vi "Keithley24XX_SR830_LakeShore336_4Probe_Resistance_Measurement_v3_Sequential.vi"() -> ()   [LabVIEW 2020]
uses:
  instr.lib/Lake Shore 336/Public/Data/Sensor Data (Single Reading).vi
  instr.lib/Stanford Research 830/Public/Data/Read (All Parameters).vi
  instr.lib/Keithley 24XX/Public/Data/Read (Single Point).vi
  instr.lib/Keithley 24XX/Keithley 24XX.lvlib
  instr.lib/Stanford Research 830/Stanford Research 830.lvlib
  instr.lib/Lake Shore 336/Lake Shore 336.lvlib
panel:
  out "Denumerated Sense":dbl
  out "SR830 X-Value":dbl
  out "SR830 Theta-Value":dbl
  out "Live Sensitivity":i16(ring)=17 items=["Auto Gain"=-1, "2 nV/fA"=0, "5 nV/fA"=1, "10 nV/fA"=2, "20 nV/fA"=3, "50 nV/fA"=4, "100 nV/fA"=5, "200 nV/fA"=6, "500 nV/fA"=7, "1 uV/pA"=8, "2 uV/pA"=9, "5 uV/pA"=10, "10 uV/pA"=11, "20 uV/pA"=12, "50 uV/pA"=13, "100 uV/pA"=14, "200 uV/pA"=15, "500 uV/pA"=16, "1 mV/nA"=17, "2 mV/nA"=18, "5 mV/nA"=19, "10 mV/nA"=20, "20 mV/nA"=21, "50 mV/nA"=22, "100 mV/nA"=23, "200 mV/nA"=24, "500 mV/mA"=25, "1 V/uA"=26]
  in  "Sensitivity (Initial Value)":i16(ring)=17 items=["Auto Gain"=-1, "2 nV/fA"=0, "5 nV/fA"=1, "10 nV/fA"=2, "20 nV/fA"=3, "50 nV/fA"=4, "100 nV/fA"=5, "200 nV/fA"=6, "500 nV/fA"=7, "1 uV/pA"=8, "2 uV/pA"=9, "5 uV/pA"=10, "10 uV/pA"=11, "20 uV/pA"=12, "50 uV/pA"=13, "100 uV/pA"=14, "200 uV/pA"=15, "500 uV/pA"=16, "1 mV/nA"=17, "2 mV/nA"=18, "5 mV/nA"=19, "10 mV/nA"=20, "20 mV/nA"=21, "50 mV/nA"=22, "100 mV/nA"=23, "200 mV/nA"=24, "500 mV/mA"=25, "1 V/uA"=26]
  in  "Dynamic Reserve (-1 = Auto)":i16(ring)=-1 items=["Auto Reserve"=-1, "High Reserve"=0, "Normal"=1, "Low Noise"=2]
  in  "Input Connection (0: Single-Ended Voltage)":u16(ring)=1 items=["Single-Ended Voltage", "Differential Voltage", "1 MOhm Current Gain", "100 MOhm Current Gain"]
  out "Input Coupling (0: AC)":u16(ring) items=["AC", "DC"]
  in  "Time Constant (8: 100ms)":u16(ring)=9 items=["10 us", "30 us", "100 us", "300 us", "1 ms", "3 ms", "10 ms", "30 ms", "100 ms", "300 ms", "1 s", "3 s", "10 s", "30 s", "100 s", "300 s", "1 ks", "3 ks", "10 ks", "30 ks"]
  in  "SR830 VISA resource name":refnum<visa-resource-name>="GPIB0::10::INSTR"
  out "Sense\nUnder":bool
  out "Sense\nOver":bool
  in  "Trigger Source (0: Internal)":u16(ring) items=["Internal", "External"]
  out "Manual Phase (0 Degree)":dbl
  out "Detection Harmonic Number":dbl=1.0
  out "External Reference Trigger (0: Sine Zero Crossing)":u16(ring) items=["Sine Zero Crossing", "TTL Rising Edge", "TTL Falling Edge"]
  in  "Internal Reference Frequency (1000 Hz)":dbl=17.0
  in  "Reference Source (1: Internal)":u16(ring)=1 items=["External", "Internal"]
  in  "Sine Output Amplitude (V)":dbl=1.0
  out "Gate\nVoltage":sgl
  out "Status":sgl
  out "Leakage \nCurrent":sgl
  in  "Temp Vs Time":enum32{"XY Graph", "Waveform (Time)"}(tab)
  out "Temp vs Time : XYGraph":cluster{"Y":dbl[], "Y":dbl[]}[](graph)
  out "Temp vs Time : TimeGraph":cluster{i32, "Sensor Data":dbl}[](graph)
  in  "Data Source (0:Kelvin)":u16(ring) items=["Kelvin", "Celsius", "Sensor Units"]
  in  "Input (0:A)":u16(ring) items=["A", "B", "C", "D"]
  in  "Serial Configuration 2":T1={"Baud Rate"=57600, "Parity"=1, "Data Bits"=7, "Stop Bits"=10, "Flow Control"=0} {"Flow Control" items=["None", "XON/XOFF", "RTS/CTS", "XON/XOFF & RTS/CTS", "DTR/DSR", "XON/XOFF & DTR/DSR"]; "Stop Bits" items=["1.0"=10, "1.5"=15, "2.0"=20]; "Data Bits" items=["7"=7, "8"=8]; "Parity" items=["None", "Odd", "Even", "Mark", "Space"]; "Baud Rate" items=["300"=300, "600"=600, "1200"=1200, "2400"=2400, "4800"=4800, "9600"=9600, "19200"=19200, "38400"=38400, "57600"=57600]}
  in  "LakeShore 336 esource name":refnum<visa-resource-name>="GPIB0::12::INSTR"
  out "dup path":path
  in  "<File Name>.txt (Don't add extension)":string
  in  "Data Save Path:":path=path "C:/Users/labpc/Documents/ProbeStation Users Data"
  in  "I_leak vs Vg":enum32{"XY Graph", "Waveform (Time)"}(tab)
  out "I_leak vs Vg : XYGraph":cluster{"Y":dbl[], "Y":dbl[]}[](graph)
  out "I_leak vs Vg : TimeGraph":cluster{dbl, "Current":sgl}[](graph)
  in  "Gate Voltage\nInitial (V)":dbl
  out "Gate Voltage\nTraversal Direction":enum16{"Upward", "Downward"}(ring)
  in  "Series Resistance \n(Apparatus Constant)":dbl=10000000.0
  in  "stop":bool
  out "Max/Min(-) \nGate Voltage (V)":dbl=80.0
  in  "Gate Voltage \nStep Size (V)":dbl=0.1
  in  "High Gate \nVoltage (V)":dbl
  in  "Low Gate \nVoltage (V)":dbl
  out "Compliance\n Level (A)":dbl=0.1
  in  "Theta vs Vg":enum32{"XY Graph", "Waveform (Time)"}(tab)
  out "Theta vs Vg : XYGraph":cluster{"Y":dbl[], "Y":dbl[]}[](graph)
  out "Theta vs Vg : TimeGraph":cluster{dbl, "Theta-Value":dbl}[](graph)
  in  "R vs Vg":enum32{"XY Graph", "Waveform (Time)"}(tab)
  out "Resistance vs Vg : XYGraph":cluster{"Y":dbl[], "Y":dbl[]}[](graph)
  out "R vs Vg : TimeGraph":cluster{dbl, dbl}[](graph)
  in  "Serial Configuration":T1={"Baud Rate"=9600, "Parity"=0, "Data Bits"=8, "Stop Bits"=10, "Flow Control"=0} {"Flow Control" items=["None", "XON/XOFF", "RTS/CTS", "XON/XOFF & RTS/CTS", "DTR/DSR", "XON/XOFF & DTR/DSR"]; "Stop Bits" items=["1.0"=10, "1.5"=15, "2.0"=20]; "Data Bits" items=["7"=7, "8"=8]; "Parity" items=["None", "Odd", "Even", "Mark", "Space"]; "Baud Rate" items=["300"=300, "600"=600, "1200"=1200, "2400"=2400, "4800"=4800, "9600"=9600, "19200"=19200]}
  in  "Keithley24XX VISA resource name":refnum<visa-resource-name>="GPIB0::21::INSTR" caption="Keithley 24XX VISA resource name"
  out "Internal Delay\nMeasurement Time (S)":dbl
  # "Lake Shore 336 Temp Contr."
  # "SR830 Lock In Amplifier"
  # "MAKE SURE THE SOURCE METER IS ON TO ENSURE NO UNINTENDED JUMPS. PROGRAM WILL KEEP SOURCE METER ON ONCE RUN."
  # "Keithley 2400 SourceMeter"
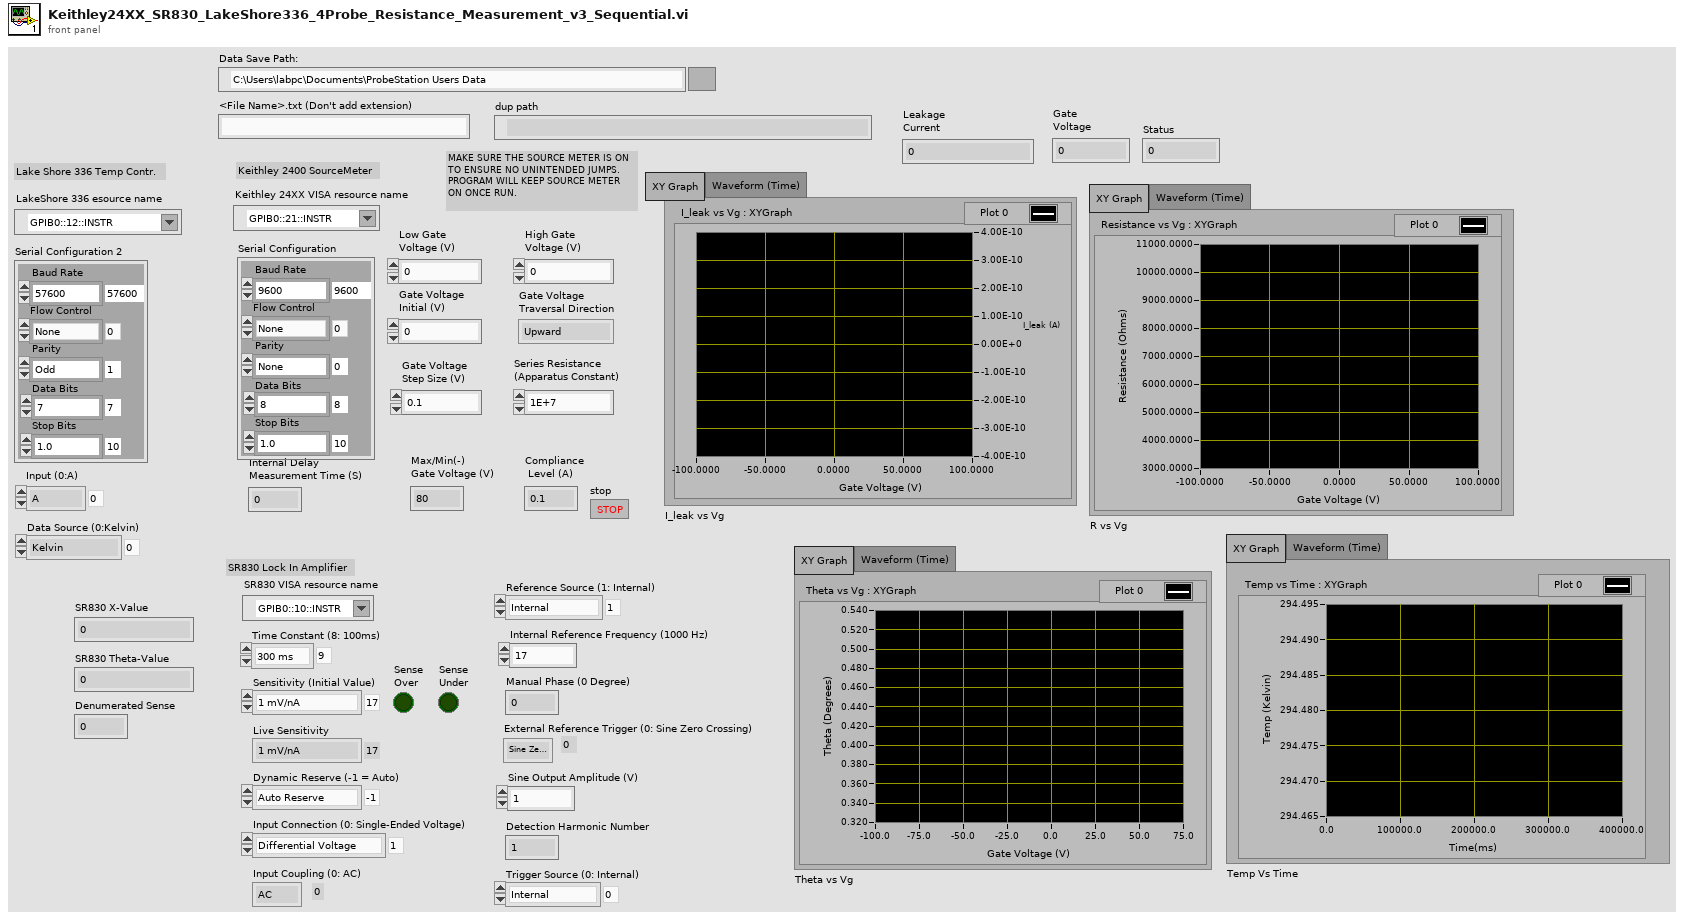
[diagram p1: front panel]
types:
  T1 = cluster{"Baud Rate":u32, "Parity":u16, "Data Bits":u16, "Stop Bits":u16, "Flow Control":u16}
  T2 = enum16{"open", "replace", "create", "open or create", "replace or create", "replace or create with confirmation"}
  T3 = cluster{"X-Value":dbl, "Y-Value":dbl, "R-Value":dbl, "Theta-Value":dbl, "Aux In 1 Value":dbl, "Aux In 2 Value":dbl, "Aux In 3 Value":dbl, "Aux In 4 Value":dbl, "Reference Frequency":dbl, "Channel 1 Display":dbl, "Channel 2 Display":dbl}
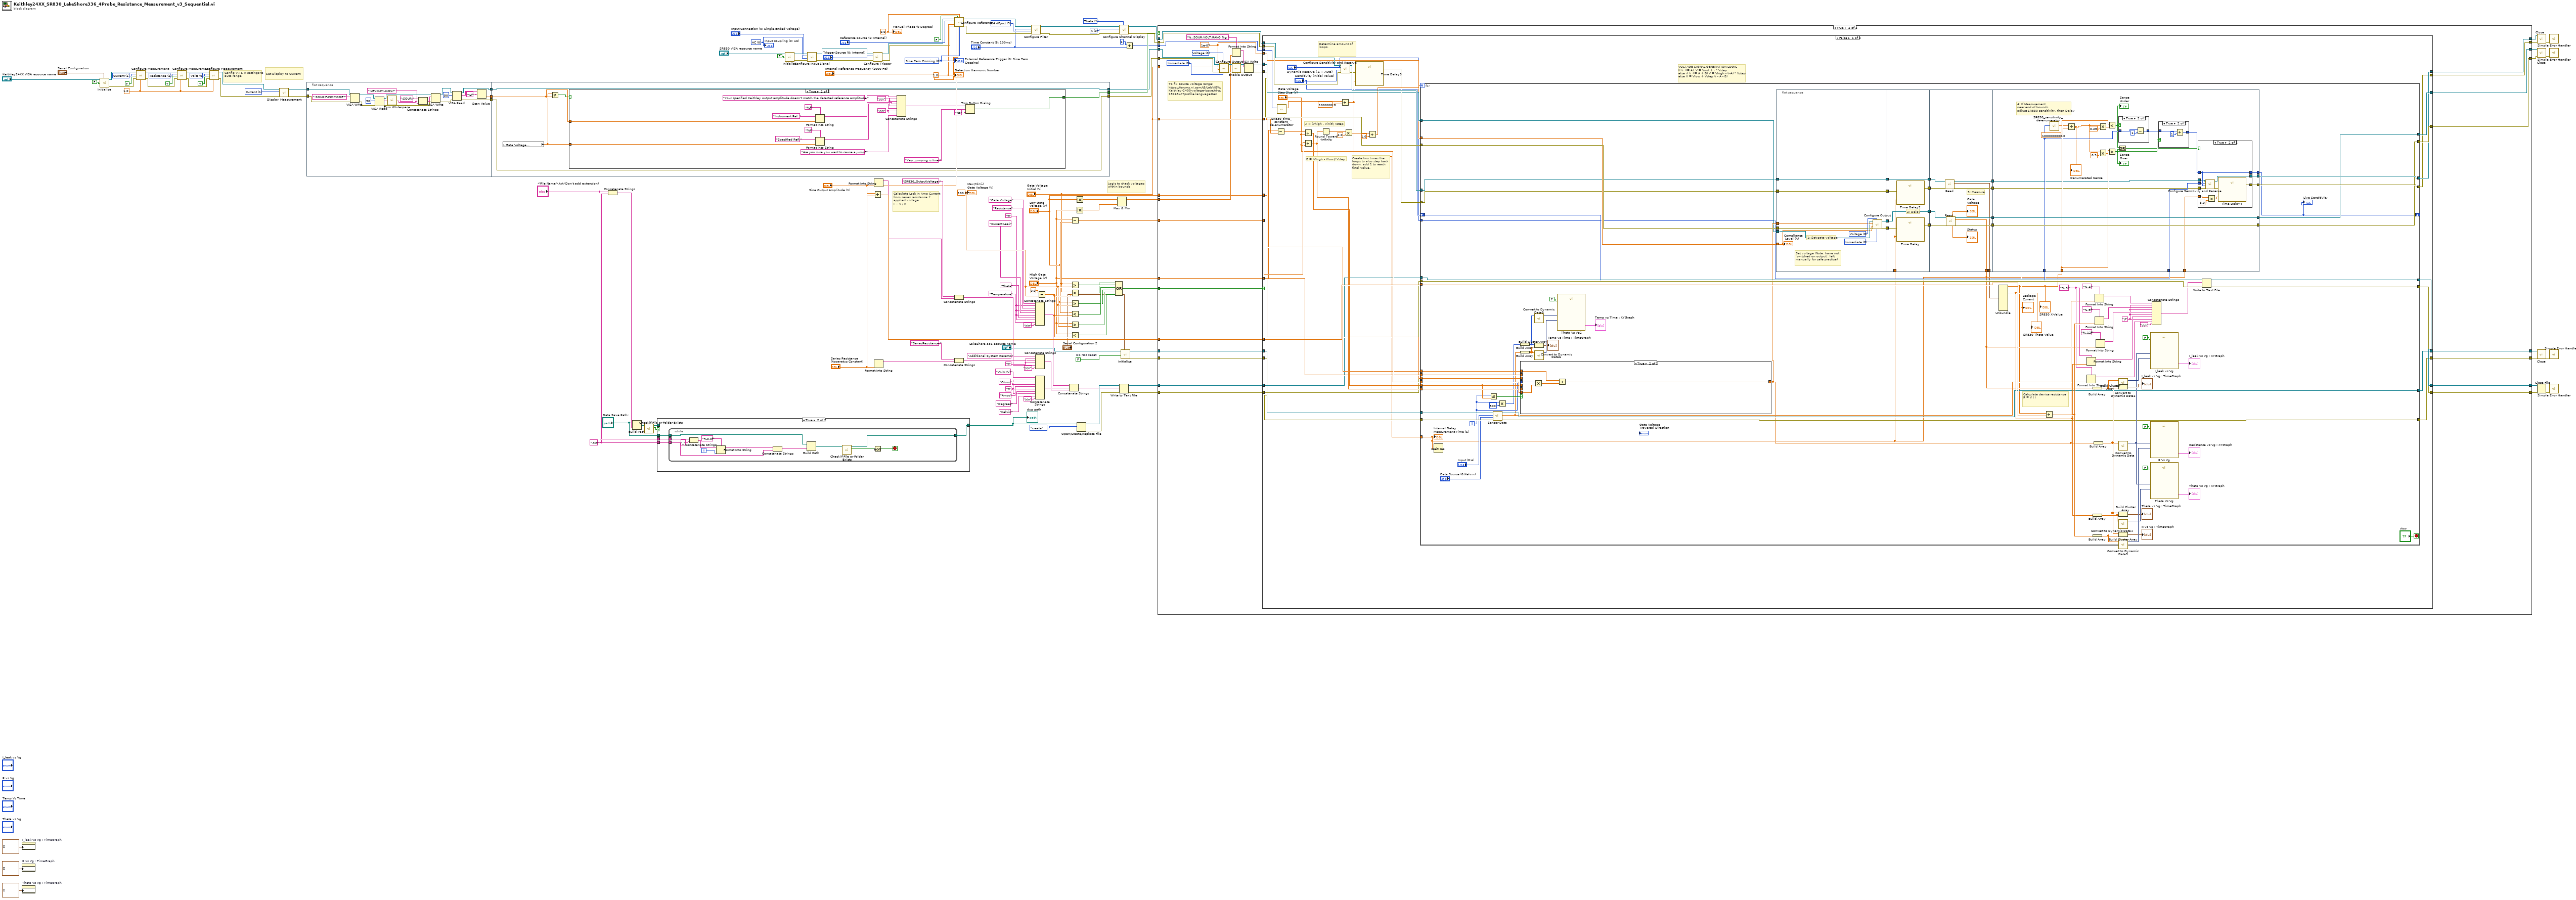
[diagram p0: block diagram]
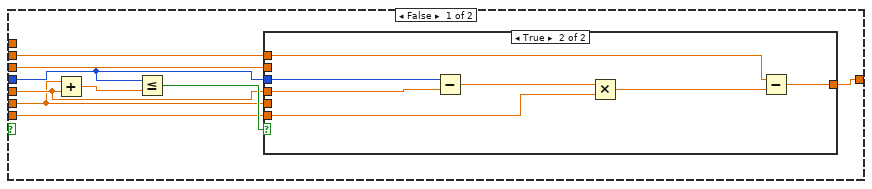
[diagram p6: hidden frame]
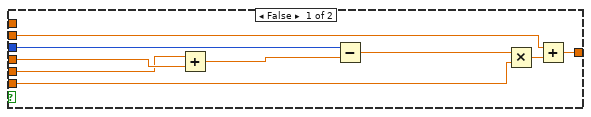
[diagram p7: hidden frame]
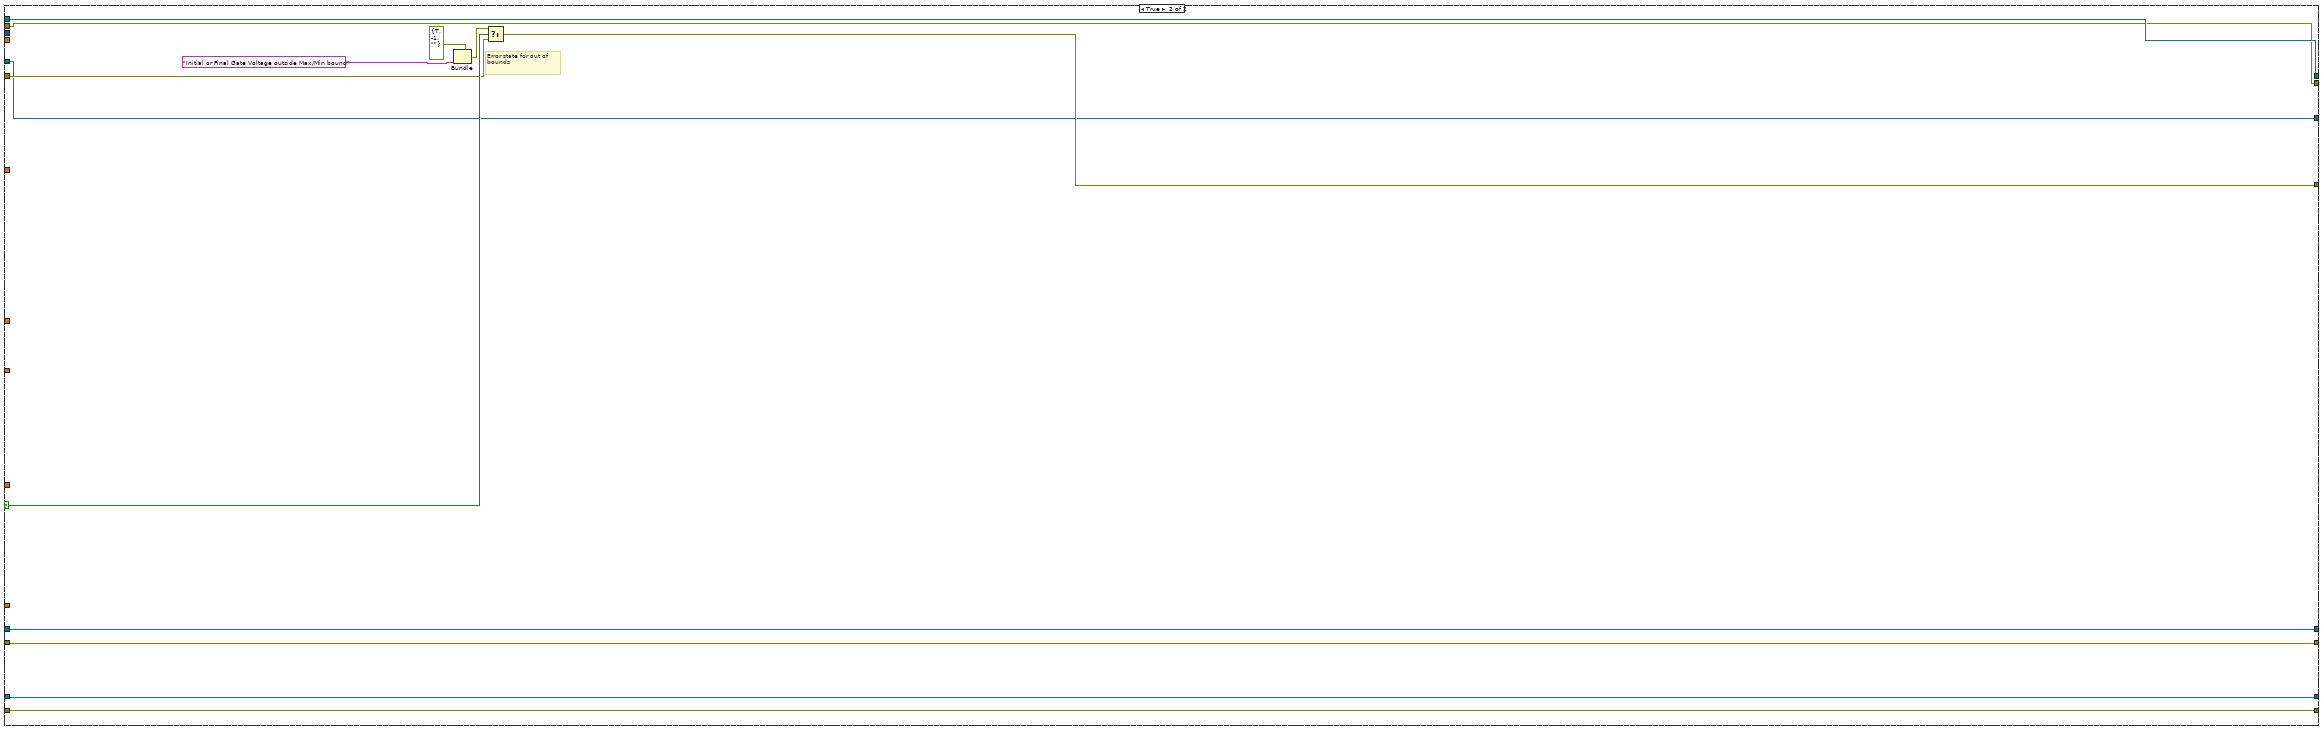
[diagram p8: hidden frame]
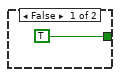
[diagram p9: hidden frame]
diagram:
  w4 = u16 3 items=["6 dB/oct", "12 dB/oct", "18 db/oct", "24 dB/oct"] ("Low Pass Filter Slope (1: 12dB/oct)")
  w31 = FALSE  # Do Not Reset
  w37 = "\t"
  w20 = "\t"
  w22 = "\t"
  w65 = ".txt"
  w72 = 1.0 ("Manual Range (1.0)")
  w96 = 0.0 ("Manual Phase (0 Degree)")
  w97 = 1.0 ("Detection Harmonic Number (1)")
  w98 = u16 0 items=["Sine Zero Crossing", "TTL Rising Edge", "TTL Falling Edge"] ("External Reference Trigger (0: Sine Zero Crossing)")
  w102 = u16 0 items=["AC", "DC"] ("Input Coupling (0: AC)")
  w84 = u16 0 items=["X", "R", "X Noise", "Aux In 1", "Aux In 2"] ("Channel 1 Display (0: X)")
  w111 = u16 1 items=["Y", "Theta", "Y Noise", "Aux In 3", "Aux In 4"] ("Channel 2 Display  (0: Y)")
  w116 = u16 1 items=["Voltage", "Current", "Resistance"] ("Displayed Measurement (0: Voltage)")
  w125 = u16 2 items=["Volts", "Current", "Resistance"] ("Function (0: Volts)")
  w129 = u16 1 items=["Volts", "Current", "Resistance"] ("Function (0: Volts)")
  w73 = 100.0
  w135 = u16 0 items=["Volts", "Current", "Resistance"] ("Function (0: Volts)")
  # "Logic to check voltages within bounds"
  # "Calculate Lock In Amp Current from series resistance + applied voltage\nI = V / R"
  # "Set Display to Current"
  # "Config V,I & R settings to auto range"
  n1 = property on="I_leak vs Vg : TimeGraph" class="WFChart (strict)"("History Data"=cluster{dbl, "Current":sgl}[] []) -> ()  [unwired: 2 in, 2 out]
  n2 = property on="R vs Vg : TimeGraph" class="WFChart (strict)"("History Data"=cluster{dbl, dbl}[] []) -> ()  [unwired: 2 in, 2 out]
  n3 = property on="Theta vs Vg : TimeGraph" class="WFChart (strict)"("History Data"=cluster{dbl, "Theta-Value":dbl}[] []) -> ()  [unwired: 2 in, 2 out]
  n4 = call "Initialize.vi"("Serial Configuration"="Serial Configuration", "Reset (True)"=FALSE, "VISA resource name"="Keithley24XX VISA resource name") -> ("error out"=w120:errorcluster, "VISA resource name out"=w121:refnum<visa-resource-name>)  [unwired: 7 in]
  n5 = call "Configure Measurement.vi"("Manual Range (1.0)"=w72, "error in (no error)"=w120, "Enable Auto Range (T:Enable)"=TRUE, "Function (0: Volts)"=w129, "VISA resource name"=w121) -> ("error out"=w127:errorcluster, "VISA resource name out"=w122:refnum<visa-resource-name>)  [unwired: 5 in]
  n6 = call "Configure Measurement.vi"("Manual Range (1.0)"=w72, "error in (no error)"=w127, "Enable Auto Range (T:Enable)"=TRUE, "Function (0: Volts)"=w125, "VISA resource name"=w122) -> ("error out"=w124:errorcluster, "VISA resource name out"=w123:refnum<visa-resource-name>)  [unwired: 5 in]
  n7 = call "Configure Measurement.vi"("Manual Range (1.0)"=w72, "error in (no error)"=w124, "Enable Auto Range (T:Enable)"=TRUE, "Function (0: Volts)"=w135, "VISA resource name"=w123) -> ("error out"=w114:errorcluster, "VISA resource name out"=w115:refnum<visa-resource-name>)  [unwired: 5 in]
  n8 = call "Display Measurement.vi"("error in (no error)"=w114, "Displayed Measurement (0: Voltage)"=w116, "VISA resource name"=w115) -> ("error out"=w10:errorcluster, "VISA resource name out"=w11:refnum<visa-resource-name>)  [unwired: 7 in]
  n9 = flat-sequence {
    tunnel: [w139] -> w14
    tunnel: [w140] -> w13
    tunnel: [w141] -> w12
    tunnel: w11 -> [w138]
    tunnel: w10 -> [w137]
    tunnel: w14 -> [w160]
    tunnel: w13 -> [w159]
    tunnel: w12 -> [w163]
    tunnel: [w160] -> w6
    tunnel: [w159] -> w8
    tunnel: [w158] -> w9
    frame #0 {
      n10 = VISA Write(VISA resource name=w138, write buffer=":SOUR:FUNC:MODE?", error in (no error)=w137) -> (VISA resource name out=w154:refnum<visa-resource-name>, error out=w157:errorcluster)  [unwired: 1 out]
      n11 = VISA Read(VISA resource name=w154, byte count=u32 50, error in (no error)=w157) -> (VISA resource name out=w149:refnum<visa-resource-name>, read buffer=w143:string, error out=w150:errorcluster)  [unwired: 1 out]
      n12 = call <vilib>:"Trim Whitespace.vi"("string"=w143) -> ("trimmed string"=w142:string)  [unwired: 1 in]
      n13 = Concatenate Strings(":SOUR:" ("string"), w142, ":LEV:IMM:AMPL?" ("string")) -> (w146:string)
      n14 = VISA Write(VISA resource name=w149, write buffer=w146, error in (no error)=w150) -> (VISA resource name out=w151:refnum<visa-resource-name>, error out=w153:errorcluster)  [unwired: 1 out]
      n15 = VISA Read(VISA resource name=w151, byte count=u32 50, error in (no error)=w153) -> (VISA resource name out=w139:refnum<visa-resource-name>, read buffer=w144:string, error out=w140:errorcluster)  [unwired: 1 out]
      n16 = Scan Value(string=w144, format string="%f") -> (value=w141:dbl)  [unwired: 1 in, 1 out]
    }
    frame #1 {
      n17 = local read "Gate Voltage\nInitial (V)"() -> (w161:dbl)
      n18 = Not Equal?(x=w161, y=w163) -> (x != y?=w162:bool)
      n19 = case shown="True" w162 {
        tunnel: [TRUE ("T button?") w171] -> w158
        tunnel: w163 -> [_ w166]
        tunnel: w161 -> [_ w165]
        frame False {
        }
        frame True {
          w169 = "\r\n"
          w167 = "\r\n"
          n20 = Format Into String(format string="%f", initial string="Instrument Ref: ", w166) -> (resulting string=w173:string)  [unwired: 1 in, 1 out]
          n21 = Format Into String(format string="%f", initial string="Specified Ref: ", w165) -> (resulting string=w172:string)  [unwired: 1 in, 1 out]
          n22 = Concatenate Strings("Your specified Keithley output amplitude doesn't match the detected reference amplitude." ("message"), w167, w167, w173, w167, w172, w169, w169, "Are you sure you want to cause a jump?" ("string")) -> (w178:string)
          n23 = Two Button Dialog(message=w178, 1:"No" ("F button name (\"Cancel\")"), 2:"Yep, jumping is fine." ("T button name (\"OK\")")) -> (T button?=w171:bool)
        }
      }
    }
  }
  n24 = Concatenate Strings("<File Name>.txt (Don't add extension)", w65) -> (w71:string)
  n25 = Build Path(base path="Data Save Path:", name or relative path=w71) -> (appended path=w70:path)
  n26 = call <vilib>:"Check if File or Folder Exists.vi"("path"=w70) -> ("file or folder exists?"=w69:bool, "dup path"=w68:path)  [unwired: 8 in, 1 out]
  n27 = case shown="True" w69 {
    tunnel: [w181 w182] -> w62
    tunnel: w68 -> [w181 _]
    tunnel: "Data Save Path:" -> [_ w183]
    tunnel: "<File Name>.txt (Don't add extension)" -> [_ w185]
    tunnel: w65 -> [_ w184]
    frame False {
    }
    frame True {
      n28 = while {
        tunnel: w185 -> [w188]
        tunnel: w184 -> [w193]
        tunnel: w183 -> [w191]
        tunnel: [w189] -> w182
        i -> [w195]
        stop <- w197 stop-if-true
        n29 = Concatenate Strings(w188, "_" ("string")) -> (w187:string)
        n30 = Format Into String(format string="%0.0f", initial string=w187, w195) -> (resulting string=w194:string)  [unwired: 1 in, 1 out]
        n31 = Concatenate Strings(w194, w193) -> (w192:string)
        n32 = Build Path(base path=w191, name or relative path=w192) -> (appended path=w190:path)
        n33 = call <vilib>:"Check if File or Folder Exists.vi"("path"=w190) -> ("file or folder exists?"=w198:bool, "dup path"=w189:path)  [unwired: 8 in, 1 out]
        n34 = Not(x=w198) -> (.not. x?=w197:bool)
      }
    }
  }
  "dup path" <- w62
  n35 = call "Initialize.vi"("Reset (True)"=FALSE, "VISA resource name"="SR830 VISA resource name") -> ("error out"=w109:errorcluster, "VISA resource name out"=w110:refnum<visa-resource-name>)  [unwired: 8 in]
  n36 = call "Configure Input Signal.vi"("error in (no error)"=w109, "Input Coupling (0: AC)"=w102, "Input Connection (0: Single-Ended Voltage)"="Input Connection (0: Single-Ended Voltage)", "VISA resource name"=w110) -> ("error out"=w93:errorcluster, "VISA resource name out"=w94:refnum<visa-resource-name>)  [unwired: 6 in]
  n37 = call "Configure Trigger.vi"("error in (no error)"=w93, "Trigger Source (0: Internal)"="Trigger Source (0: Internal)", "VISA resource name"=w94) -> ("error out"=w91:errorcluster, "VISA resource name out"=w92:refnum<visa-resource-name>)  [unwired: 7 in]
  n38 = Divide(x="Sine Output Amplitude (V)", y="Series Resistance \n(Apparatus Constant)") -> (x/y=w90:dbl)
  n39 = Format Into String("Sine Output Amplitude (V)") -> (resulting string=w54:string)  [unwired: 3 in, 1 out]
  n40 = Format Into String("Series Resistance \n(Apparatus Constant)") -> (resulting string=w55:string)  [unwired: 3 in, 1 out]
  n41 = call "Configure Reference.vi"("VISA resource name"=w92, "Auto Phase (T: Enabled)"=FALSE, "Manual Phase (0 Degree)"=w96, "Reference Source (1: Internal)"="Reference Source (1: Internal)", "Sine Output Amplitude (1 V)"="Sine Output Amplitude (V)", "Detection Harmonic Number (1)"=w97, "error in (no error)"=w91, "Internal Reference Frequency (1000 Hz)"="Internal Reference Frequency (1000 Hz)", "External Reference Trigger (0: Sine Zero Crossing)"=w98) -> ("VISA resource name out"=w99:refnum<visa-resource-name>, "error out"=w100:errorcluster)  [unwired: 5 in]
  n42 = Concatenate Strings("SR830_OutputVoltage:" ("string"), w54) -> (w35:string)
  n43 = Concatenate Strings("SeriesResistance:" ("string"), w55) -> (w36:string)
  n44 = call "Configure Filter.vi"("error in (no error)"=w100, "Low Pass Filter Slope (1: 12dB/oct)"=w4, "Time Constant (8: 100ms)"="Time Constant (8: 100ms)", "VISA resource name"=w99) -> ("error out"=w118:errorcluster, "VISA resource name out"=w117:refnum<visa-resource-name>)  [unwired: 6 in]
  n45 = Concatenate Strings("Gate Voltage" ("string"), w22, "Resistance" ("string"), w22, "Current Leak" ("string"), w22, "Theta" ("string"), w22, "Temperature" ("string"), "\r\n") -> (w49:string)
  n46 = Concatenate Strings("Volts (V)" ("string"), w20, "Ohms" ("string"), w20, "Amps" ("string"), w20, "Degrees" ("string"), w20, "Kelvin" ("string"), "\r\n") -> (w48:string)
  n47 = Concatenate Strings("Additional System Params:" ("string"), w37, w36, w37, w35, "\r\n") -> (w38:string)
  n48 = Subtract(x=0.0, y=w73) -> (x-y=w78:dbl)
  n49 = Concatenate Strings(w49, w48, w38) -> (w33:string)
  n50 = Subtract(x="High Gate \nVoltage (V)", y="Low Gate \nVoltage (V)") -> (x-y=w74:dbl)
  n51 = Greater?(x="Gate Voltage\nInitial (V)", y=w73) -> (0:w77:bool)
  n52 = Less?(x="Gate Voltage\nInitial (V)", y=w78) -> (x < y?=w76:bool)
  n53 = Greater?(x="Low Gate \nVoltage (V)", y=w73) -> (0:w81:bool)
  n54 = Less?(x="Low Gate \nVoltage (V)", y=w78) -> (x < y?=w82:bool)
  n55 = Greater?(x="High Gate \nVoltage (V)", y=w73) -> (0:w80:bool)
  n56 = Less?(x="High Gate \nVoltage (V)", y=w78) -> (x < y?=w79:bool)
  n57 = Absolute Value(x="Low Gate \nVoltage (V)") -> (abs(x)=w18:dbl)
  n58 = Absolute Value(x="High Gate \nVoltage (V)") -> (abs(x)=w17:dbl)
  n59 = Open/Create/Replace File(file path (use dialog)=w62, operation (0:open)=T2."create") -> (refnum out=w63:refnum<file>, error out=w61:errorcluster)  [unwired: 4 in, 1 out]
  n60 = Compound Arithmetic op=OR(w76, w77, w82, w81, w80, w79) -> (w75:bool)
  n61 = Max & Min(x=w18, y=w17) -> (max(x,y)=w5:dbl)  [unwired: 1 out]
  n62 = Write to Text File(file (use dialog)=w63, text=w33, error in=w61) -> (refnum out=w59:refnum<file>, error out=w58:errorcluster)  [unwired: 1 in, 1 out]
  n63 = call "Configure Channel Display.vi"("Channel 2 Display  (0: Y)"=w111, "error in (no error)"=w118, "Channel 1 Display (0: X)"=w84, "VISA resource name"=w117) -> ("error out"=w107:errorcluster, "VISA resource name out"=w108:refnum<visa-resource-name>)  [unwired: 6 in]
  n64 = call "Initialize.vi"("Serial Configuration"="Serial Configuration 2", "Reset (True)"=w31, "VISA resource name"="LakeShore 336 esource name") -> ("error out"=w26:errorcluster, "VISA resource name out"=w25:refnum<visa-resource-name>)  [unwired: 7 in]
  n65 = Add(x=u16 1, y="Time Constant (8: 100ms)") -> (x+y=w1:u16)
  n66 = case shown="True" w9 {
    tunnel: [w206 w242] -> w133
    tunnel: [w205 w241] -> w132
    tunnel: w108 -> [w204 w240]
    tunnel: w107 -> [w203 w239]
    tunnel: [w204 w238] -> w106
    tunnel: [w203 w237] -> w105
    tunnel: w90 -> [_ w236]
    tunnel: w75 -> [_ w235]
    tunnel: w74 -> [_ w234]
    tunnel: w59 -> [w202 w233]
    tunnel: w58 -> [w201 w232]
    tunnel: [w202 w231] -> w57
    tunnel: [w201 w230] -> w56
    tunnel: [w199 w229] -> w28
    tunnel: [w200 w228] -> w27
    tunnel: w26 -> [w199 w227]
    tunnel: w25 -> [w200 w226]
    tunnel: "Low Gate \nVoltage (V)" -> [_ w225]
    tunnel: "High Gate \nVoltage (V)" -> [_ w224]
    tunnel: "Gate Voltage\nInitial (V)" -> [_ w223]
    tunnel: w8 -> [w205 w215]
    tunnel: "Gate Voltage\nInitial (V)" -> [_ w214]
    tunnel: w6 -> [w206 w213]
    tunnel: w5 -> [_ w211]
    tunnel: w1 -> [_ w207]
    frame False {
    }
    frame True {
      w217 = u16 0 items=["Immediate", "Triggered"] ("Output Type  (0: Immediate)")
      w210 = 1e-07 ("Compliance  Level (0.1)")
      w216 = u16 0 items=["Voltage", "Current"] ("Source Mode  (0: Voltage)")
      # "To fix source voltage range:\nhttps://forums.ni.com/t5/LabVIEW/Keithley-2400-voltage-Issue/td-p/1926347?profile.language=en"
      n67 = call "Configure Output.vi"("Output Type  (0: Immediate)"=w217, "Source Mode  (0: Voltage)"=w216, "error in (no error)"=w215, "Compliance  Level (0.1)"=w210, "Output Level (0)"=w214, "VISA resource name"=w213) -> ("error out"=w222:errorcluster, "VISA resource name out"=w221:refnum<visa-resource-name>)  [unwired: 4 in]
      n68 = Format Into String(format string="%.;SOUR:VOLT:RANG %g ", w211) -> (resulting string=w218:string)  [unwired: 2 in, 1 out]
      n69 = call "Enable Output.vi"("error in (no error)"=w222, "VISA resource name"=w221) -> ("error out"=w220:errorcluster, "VISA resource name out"=w219:refnum<visa-resource-name>)  [unwired: 8 in]
      n70 = VISA Write(VISA resource name=w219, write buffer=w218, error in (no error)=w220) -> (VISA resource name out=w208:refnum<visa-resource-name>, error out=w209:errorcluster)  [unwired: 1 out]
      n71 = case shown="False" w235 {
        selector: w235 -> [_ w488]
        tunnel: w209 -> [w282 w487]
        tunnel: w208 -> [w250 w482]
        tunnel: [w281 w482] -> w242
        tunnel: [w280 w483] -> w241
        tunnel: w240 -> [w275 w481]
        tunnel: w239 -> [w276 w480]
        tunnel: [w278 w481] -> w238
        tunnel: [w277 w480] -> w237
        tunnel: w236 -> [w273 _]
        tunnel: w234 -> [w268 _]
        tunnel: w225 -> [w261 _]
        tunnel: w224 -> [w262 _]
        tunnel: w223 -> [w264 _]
        tunnel: w233 -> [w258 w479]
        tunnel: w232 -> [w257 w478]
        tunnel: [w256 w479] -> w231
        tunnel: [w255 w478] -> w230
        tunnel: [w252 w476] -> w229
        tunnel: [w251 w477] -> w228
        tunnel: w227 -> [w254 w476]
        tunnel: w226 -> [w253 w477]
        tunnel: w210 -> [w249 _]
        tunnel: w207 -> [w248 _]
        frame False {
          # "VOLTAGE SIGNAL GENERATION LOGIC\nIf (i <= A), V = Vinit + i * Vstep\nelse if (i <= A + B) V = Vhigh - (i-A) * Vstep\nelse V = Vlow + Vstep (i - A - B)"
          # "B = (Vhigh - Vlow)/ Vstep"
          # "A = (Vhigh - Vinit)/ Vstep"
          # "Create two times the loops to also step back down, add 1 to reach final value."
          # "Determine amount of loops,"
          n72 = Subtract(x=w262, y=w264) -> (x-y=w267:dbl)
          n73 = call "SR830_time_constant_de-enumerator.vi"("Time Constant (8: 100ms)"=w248) -> ("Time Constant (us)"=w246:dbl)  [unwired: 10 in]
          n74 = Divide(x=w267, y="Gate Voltage \nStep Size (V)") -> (x/y=w265:dbl)
          n75 = Divide(x=w268, y="Gate Voltage \nStep Size (V)") -> (x/y=w263:dbl)
          n76 = Round Toward -Infinity(1:w263) -> (0:w271:dbl)
          n77 = call "Configure Sensitivity and Reserve.vi"("error in (no error)"=w276, "Sensitivity (-1: Auto gain)"="Sensitivity (Initial Value)", "Dynamic Reserve (-1: Auto Reserve)"="Dynamic Reserve (-1 = Auto)", "VISA resource name"=w275) -> ("error out"=w259:errorcluster, "VISA resource name out"=w274:refnum<visa-resource-name>)  [unwired: 6 in]
          n78 = Divide(x=w246, y=1000000.0) -> (x/y=w245:dbl)
          n79 = Multiply(x=w271, y=2.0) -> (x*y=w270:dbl)
          n80 = call "Time Delay3"("error in (no error)"=w259, "Delay Time (s)"=w245) -> ("error out"=w260:errorcluster)  [unwired: 9 in]
          n81 = Add(x=w270, y=1.0) -> (x+y=w269:dbl)
          n82 = for {
            N: w269 -> [_]
            tunnel: w250 -> [w308]
            tunnel: w282 -> [w311]
            tunnel: [w289] -> w281
            tunnel: [w291] -> w280
            tunnel: [w296] -> w278
            tunnel: [w295] -> w277
            tunnel: w274 -> [w297]
            tunnel: w260 -> [w302]
            tunnel: w273 -> [w371]
            tunnel: "Gate Voltage \nStep Size (V)" -> [w353]
            tunnel: w265 -> [w351]
            tunnel: w264 -> [w354]
            tunnel: w263 -> [w352]
            tunnel: w262 -> [w350]
            tunnel: w261 -> [w349]
            tunnel: w258 -> [w348]
            tunnel: w257 -> [w347]
            tunnel: [w346] -> w256
            tunnel: [w345] -> w255
            tunnel: w254 -> [w328]
            tunnel: w253 -> [w327]
            tunnel: [w326] -> w252
            tunnel: [w325] -> w251
            tunnel: w249 -> [w310]
            tunnel: w245 -> [w285]
            shift-right: [w284] -> _
            shift-left: "Sensitivity (Initial Value)" -> [w287]
            tunnel: "Dynamic Reserve (-1 = Auto)" -> [w286]
            i -> [w319]
            stop <- "stop" stop-if-true
            w316 = "%.3f" ("format string")
            w313 = "\t"
            # "Calculate device resistance\nR = V / I"
            n83 = Wait (ms)(milliseconds to wait=w285) -> ()  [unwired: 1 out]
            n84 = Less Or Equal?(x=w319, y=w351) -> (x <= y?=w355:bool)
            n85 = call-poly "Sensor Data.vi"("error in (no error)"=w328, "Data Source (0:Kelvin)"="Data Source (0:Kelvin)", "Input (0:A)"="Input (0:A)", "VISA resource name"=w327) -> ("error out"=w326:errorcluster, "Sensor Data"=w315:dbl, "VISA resource name out"=w325:refnum<visa-resource-name>)  [unwired: 5 in]
            n86 = Multiply(x=w319, y=500) -> (x*y=w317:i32)
            n87 = Build Array(w317) -> (w329:i32[])
            n88 = Build Array(w315) -> (w321:dbl[])
            n89 = case shown="True" w355 {
              tunnel: [w452 w471] -> w309
              tunnel: w354 -> [_ w474]
              tunnel: w319 -> [w449 w475]
              tunnel: w353 -> [w450 w472]
              tunnel: w352 -> [w446 _]
              tunnel: w351 -> [w448 _]
              tunnel: w350 -> [w451 _]
              tunnel: w349 -> [w447 _]
              frame False {
                n90 = Add(x=w446, y=w448) -> (x+y=w453:dbl)
                n91 = Less Or Equal?(x=w449, y=w453) -> (x <= y?=w454:bool)
                n92 = case shown="True" w454 {
                  tunnel: [w460 w469] -> w452
                  tunnel: w451 -> [_ w470]
                  tunnel: w450 -> [w462 w467]
                  tunnel: w449 -> [w457 w466]
                  tunnel: w448 -> [w456 w465]
                  tunnel: w447 -> [w463 _]
                  tunnel: w446 -> [w455 _]
                  frame False {
                    n93 = Add(x=w455, y=w456) -> (x+y=w458:dbl)
                    n94 = Subtract(x=w457, y=w458) -> (x-y=w459:dbl)
                    n95 = Multiply(x=w459, y=w462) -> (x*y=w461:dbl)
                    n96 = Add(x=w463, y=w461) -> (x+y=w460:dbl)
                  }
                  frame True {
                    n97 = Subtract(x=w466, y=w465) -> (x-y=w468:dbl)
                    n98 = Multiply(x=w468, y=w467) -> (x*y=w464:dbl)
                    n99 = Subtract(x=w470, y=w464) -> (x-y=w469:dbl)
                  }
                }
              }
              frame True {
                n100 = Multiply(x=w475, y=w472) -> (x*y=w473:dbl)
                n101 = Add(x=w474, y=w473) -> (x+y=w471:dbl)
              }
            }
            n102 = call "Convert to Dynamic Data5"("Array"=w329) -> ("Dynamic Data Type"=w330:dynamicdata)  [unwired: 3 in]
            n103 = Build Cluster Array(w329, w321) -> (→"Temp vs Time : TimeGraph":cluster{i32, "Sensor Data":dbl}[])
            n104 = call "Convert to Dynamic Data6"("Array"=w321) -> ("Dynamic Data Type"=w322:dynamicdata)  [unwired: 3 in]
            n105 = call "Theta Vs Vg2"("Reset"=FALSE, "Y Input"=w322, "X Input"=w330) -> ("XY Graph"=→"Temp vs Time : XYGraph":cluster{"X":dbl[], "Y":dbl[]}[])  [unwired: 7 in, 1 out]
            n106 = flat-sequence {
              tunnel: w311 -> [w380]
              tunnel: w310 -> [w377]
              tunnel: w309 -> [w379]
              tunnel: w308 -> [w378]
              tunnel: [w376] -> w307
              tunnel: [w375] -> w305
              tunnel: w297 -> [w373]
              tunnel: w302 -> [w374]
              tunnel: [w374] -> w300
              tunnel: [w373] -> w298
              tunnel: w307 -> [w389]
              tunnel: [w389] -> w306
              tunnel: w305 -> [w385]
              tunnel: [w384] -> w304
              tunnel: [w386] -> w301
              tunnel: w300 -> [w387]
              tunnel: [w388] -> w299
              tunnel: w298 -> [w388]
              tunnel: w285 -> [w383]
              tunnel: w306 -> [w398]
              tunnel: w304 -> [w397]
              tunnel: [w399] -> w303
              tunnel: w301 -> [w395]
              tunnel: w299 -> [w396]
              tunnel: [w394] -> w294
              tunnel: [w393] -> w293
              tunnel: [w392] -> w292
              tunnel: [w391] -> w290
              tunnel: [w390] -> w288
              tunnel: [w408] -> w296
              tunnel: [w406] -> w295
              tunnel: w294 -> [w409]
              tunnel: w293 -> [w407]
              tunnel: w292 -> [w424]
              tunnel: [w424] -> w291
              tunnel: w290 -> [w423]
              tunnel: [w423] -> w289
              tunnel: w283 -> [w420]
              tunnel: w287 -> [w417]
              tunnel: [w414] -> w284
              tunnel: w286 -> [w410]
              tunnel: w285 -> [w405]
              frame #0 {
                w382 = u16 0 items=["Immediate", "Triggered"] ("Output Type  (0: Immediate)")
                w381 = u16 0 items=["Voltage", "Current"] ("Source Mode  (0: Voltage)")
                # "Set voltage (Note, have not 'switched on output', left manually for safe practise)"
                # "1: Set gate voltage"
                n107 = call "Configure Output.vi"("Output Type  (0: Immediate)"=w382, "Source Mode  (0: Voltage)"=w381, "error in (no error)"=w380, "Compliance  Level (0.1)"=w377, "Output Level (0)"=w379, "VISA resource name"=w378) -> ("error out"=w375:errorcluster, "VISA resource name out"=w376:refnum<visa-resource-name>)  [unwired: 4 in]
                "Compliance\n Level (A)" <- w377
              }
              frame #1 {
                # "2: Delay"
                n108 = call "Time Delay2"("error in (no error)"=w387, "Delay Time (s)"=w383) -> ("error out"=w386:errorcluster)  [unwired: 9 in]
                n109 = call "Time Delay"("error in (no error)"=w385, "Delay Time (s)"=w383) -> ("error out"=w384:errorcluster)  [unwired: 9 in]
              }
              frame #2 {
                # "3: Measure"
                n110 = call-poly "Read.vi"("error in (no error)"=w395, "VISA resource name"=w396) -> ("error out"=w393:errorcluster, "Parameter Values"=w390:T3, "VISA resource name out"=w394:refnum<visa-resource-name>)  [unwired: 7 in]
                n111 = call-poly "Read.vi"("VISA resource name"=w398, "error in (no error)"=w397) -> ("Voltage"=→"Gate\nVoltage":sgl, "VISA resource name out"=w391:refnum<visa-resource-name>, "Current"=w399:sgl, "Status"=→"Status":sgl, "error out"=w392:errorcluster)  [unwired: 7 in, 2 out]
              }
              frame #3 {
                # "4: If Measurement\nnear end of bounds, \nadjust SR830 sensitivity, then Delay"
                n112 = call "SR830_sensitivity_de-enumerator.vi"("Sensitivity (Initial Value)"=w417) -> ("Sensitivity (nV/fA)"=w404:dbl)  [unwired: 10 in]
                n113 = Divide(x=w404, y=1000000000.0) -> (x/y=w402:dbl)
                "Denumerated Sense" <- w402
                n114 = Multiply(x=w402, y=0.25) -> (x*y=w418:dbl)
                n115 = Multiply(x=w402, y=0.9) -> (x*y=w419:dbl)
                n116 = Less?(x=w420, y=w418) -> (x < y?=w413:bool)
                "Sense\nUnder" <- w413
                n117 = Greater?(x=w420, y=w419) -> (0:w412:bool)
                "Sense\nOver" <- w412
                n118 = Or(x=w413, y=w412) -> (x .or. y?=w411:bool)
                n119 = case shown="True" w413 {
                  tunnel: w417 -> [w442 w445]
                  tunnel: [w442 w443] -> w416
                  frame False {
                  }
                  frame True {
                    n120 = Subtract(x=w445, y=i16 1) -> (x-y=w443:i16)
                  }
                }
                n121 = case shown="True" w412 {
                  tunnel: w416 -> [w438 w441]
                  tunnel: [w438 w439] -> w415
                  frame False {
                  }
                  frame True {
                    n122 = Add(x=w441, y=i16 1) -> (x+y=w439:i16)
                  }
                }
                n123 = case shown="True" w411 {
                  tunnel: w415 -> [w427 w436]
                  tunnel: [w427 w436] -> w414
                  tunnel: w410 -> [_ w437]
                  tunnel: w409 -> [w426 w435]
                  tunnel: [w426 w434] -> w408
                  tunnel: w407 -> [w425 w433]
                  tunnel: [w425 w431] -> w406
                  tunnel: w405 -> [_ w430]
                  frame False {
                  }
                  frame True {
                    n124 = call "Configure Sensitivity and Reserve.vi"("error in (no error)"=w433, "Sensitivity (-1: Auto gain)"=w436, "Dynamic Reserve (-1: Auto Reserve)"=w437, "VISA resource name"=w435) -> ("error out"=w432:errorcluster, "VISA resource name out"=w434:refnum<visa-resource-name>)  [unwired: 6 in]
                    n125 = Multiply(x=w430, y=3.0) -> (x*y=w429:dbl)
                    n126 = call "Time Delay4"("error in (no error)"=w432, "Delay Time (s)"=w429) -> ("error out"=w431:errorcluster)  [unwired: 9 in]
                  }
                }
              }
            }
            n127 = Unbundle(w288) -> ("X-Value"=w283:dbl, "Theta-Value"=w338:dbl)  [unwired: 9 out]
            "SR830 Theta-Value" <- w338
            "SR830 X-Value" <- w283
            n128 = Divide(x=w283, y=w371) -> (x/y=w339:dbl)
            n129 = Format Into String(format string=w316, w338) -> (resulting string=w341:string)  [unwired: 2 in, 1 out]
            n130 = Format Into String(format string=w316, w315) -> (resulting string=w312:string)  [unwired: 2 in, 1 out]
            n131 = Build Array(w303) -> (w368:sgl[])
            n132 = Build Array(w338) -> (w364:dbl[])
            n133 = Build Array(w339) -> (w366:dbl[])
            n134 = Build Array(w309) -> (w332:dbl[])
            n135 = Format Into String(format string="%.4f", w309) -> (resulting string=w344:string)  [unwired: 2 in, 1 out]
            n136 = Format Into String(format string="%.9f", w339) -> (resulting string=w343:string)  [unwired: 2 in, 1 out]
            n137 = Format Into String(format string="%.12f", w303) -> (resulting string=w342:string)  [unwired: 2 in, 1 out]
            n138 = call "Convert to Dynamic Data2"("Array"=w368) -> ("Dynamic Data Type"=w367:dynamicdata)  [unwired: 3 in]
            n139 = Build Cluster Array(w332, w368) -> (→"I_leak vs Vg : TimeGraph":cluster{dbl, "Current":sgl}[])
            n140 = Build Cluster Array(w332, w364) -> (→"Theta vs Vg : TimeGraph":cluster{dbl, "Theta-Value":dbl}[])
            n141 = call "Convert to Dynamic Data4"("Array"=w364) -> ("Dynamic Data Type"=w363:dynamicdata)  [unwired: 3 in]
            n142 = Build Cluster Array(w332, w366) -> (→"R vs Vg : TimeGraph":cluster{dbl, dbl}[])
            n143 = call "Convert to Dynamic Data3"("Array"=w366) -> ("Dynamic Data Type"=w365:dynamicdata)  [unwired: 3 in]
            n144 = call "Convert to Dynamic Data"("Array"=w332) -> ("Dynamic Data Type"=w331:dynamicdata)  [unwired: 3 in]
            n145 = call "I_leak vs Vg"("Reset"=FALSE, "Y Input"=w367, "X Input"=w331) -> ("XY Graph"=→"I_leak vs Vg : XYGraph":cluster{"X":dbl[], "Y":dbl[]}[])  [unwired: 7 in, 1 out]
            n146 = call "R Vs Vg"("Reset"=FALSE, "Y Input"=w365, "X Input"=w331) -> ("XY Graph"=→"Resistance vs Vg : XYGraph":cluster{"X":dbl[], "Y":dbl[]}[])  [unwired: 7 in, 1 out]
            n147 = call "Theta Vs Vg"("Reset"=FALSE, "Y Input"=w363, "X Input"=w331) -> ("XY Graph"=→"Theta vs Vg : XYGraph":cluster{"X":dbl[], "Y":dbl[]}[])  [unwired: 7 in, 1 out]
            n148 = Concatenate Strings(w344, w313, w343, w313, w342, w313, w341, w313, w312, "\r\n") -> (w340:string)
            n149 = Write to Text File(file (use dialog)=w348, text=w340, error in=w347) -> (refnum out=w346:refnum<file>, error out=w345:errorcluster)  [unwired: 1 in, 1 out]
            "Internal Delay\nMeasurement Time (S)" <- w285
            "Leakage \nCurrent" <- w303
            "Live Sensitivity" <- w284
          }
        }
        frame True {
          # "Error state for out of bounds"
          n150 = Bundle(cluster=errorcluster {"status"=TRUE, "code"=-1, "source"=""} ("error constant"), "source"="Initial or Final Gate Voltage outside Max/Min bound") -> (w484:errorcluster)  [unwired: 2 in]
          n151 = Select(t=w484, s=w488, f=w487) -> (s? t:f=w483:errorcluster)
        }
      }
    }
  }
  n152 = call "Close.vi"("error in (no error)"=w105, "VISA resource name"=w106) -> ("error out"=w119:errorcluster)  [unwired: 9 in]
  n153 = call "Close.vi"("error in (no error)"=w132, "VISA resource name"=w133) -> ("error out"=w131:errorcluster)  [unwired: 9 in]
  n154 = call "Close.vi"("error in (no error)"=w28, "VISA resource name"=w27) -> ("error out"=w29:errorcluster)  [unwired: 9 in]
  n155 = Close File(refnum=w57, error in=w56) -> (error out=w60:errorcluster)  [unwired: 1 out]
  n156 = call <vilib>:"Simple Error Handler.vi"("error in (no error)"=w119) -> ()  [unwired: 4 in, 5 out]
  n157 = call <vilib>:"Simple Error Handler.vi"("error in (no error)"=w131) -> ()  [unwired: 4 in, 5 out]
  n158 = call <vilib>:"Simple Error Handler.vi"("error in (no error)"=w29) -> ()  [unwired: 4 in, 5 out]
  n159 = call <vilib>:"Simple Error Handler.vi"("error in (no error)"=w60) -> ()  [unwired: 4 in, 5 out]
  "Max/Min(-) \nGate Voltage (V)" <- w73
  "Input Coupling (0: AC)" <- w102
  "External Reference Trigger (0: Sine Zero Crossing)" <- w98
  "Detection Harmonic Number" <- w97
  "Manual Phase (0 Degree)" <- w96
